vi "Write DAT.vi"   [LabVIEW 2016, in "LV-Data.DAT.lvclass"]
uses:
  LV-Data.DAT.lvclass
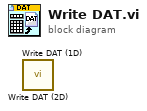
[diagram p0: block diagram]
diagram:
  n1 = call "Write DAT (2D).vi"() -> ()  [unwired: 10 in, 2 out]
  n2 = call "Write DAT (1D).vi"() -> ()  [unwired: 10 in, 2 out]
